vi "timerRunNew.vi"() -> ()   [LabVIEW 2012]
uses:
  <vilib>/addons/database/Connection.llb/DB Tools Open Connec (Path).vi
  <vilib>/addons/database/Connection.llb/Conn Execute.vi
  <vilib>/addons/database/Recordset.llb/Rec Fetch Recordset Data (R).vi
  <vilib>/addons/database/Recordset.llb/Rec Destroy - Connection.vi
  <vilib>/addons/database/_DB Variant To Data/Database Variant To Data.xnode
  <vilib>/addons/database/NI_Database_API.lvlib
panel:
  out "error out 4":errorcluster
  out "error out 3":errorcluster
  out "recordset data 3":variant[][](array[variant])
  out "error out 2":errorcluster
  out "recordset data 2":variant[][](array[variant])
  out "error out":errorcluster
  out "recordset data":variant[][](array[variant])
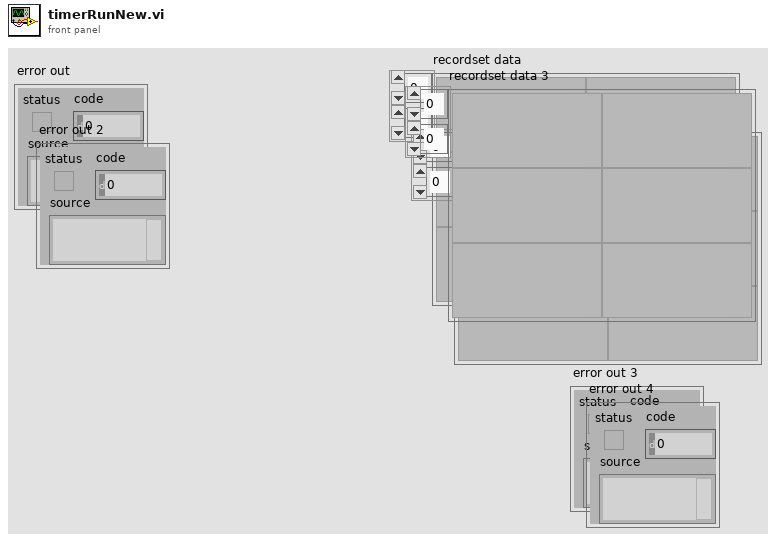
[diagram p1: front panel]
types:
  T1 = typedef "NI_Database_API.lvlib/Conn ObjectReference.ctl" = refnum<k1>
  T2 = typedef "NI_Database_API.lvlib/Rec ObjectReference.ctl" = refnum<k1>
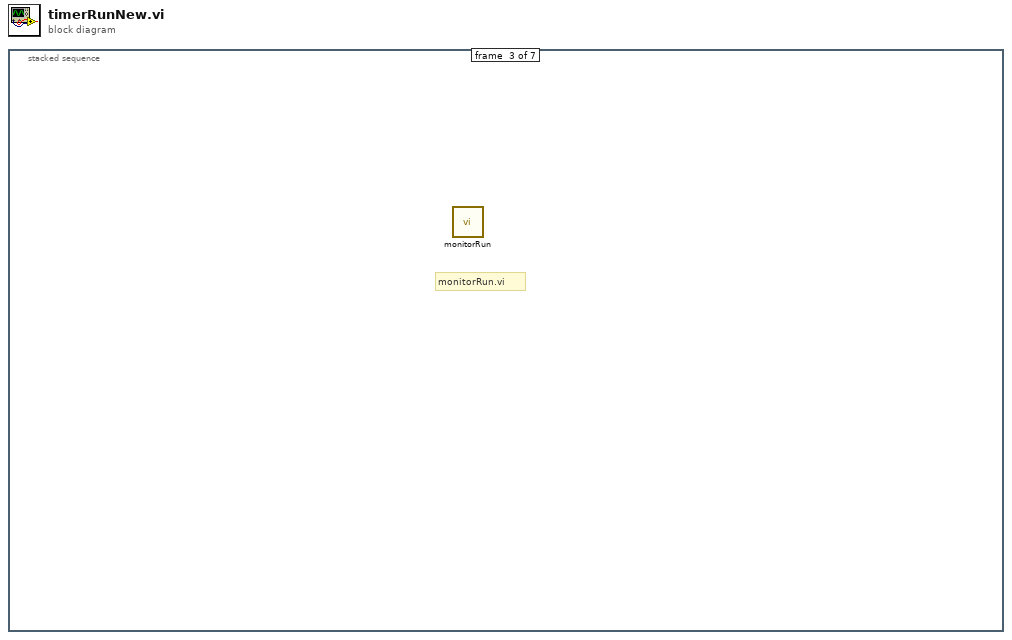
[diagram p0: block diagram]
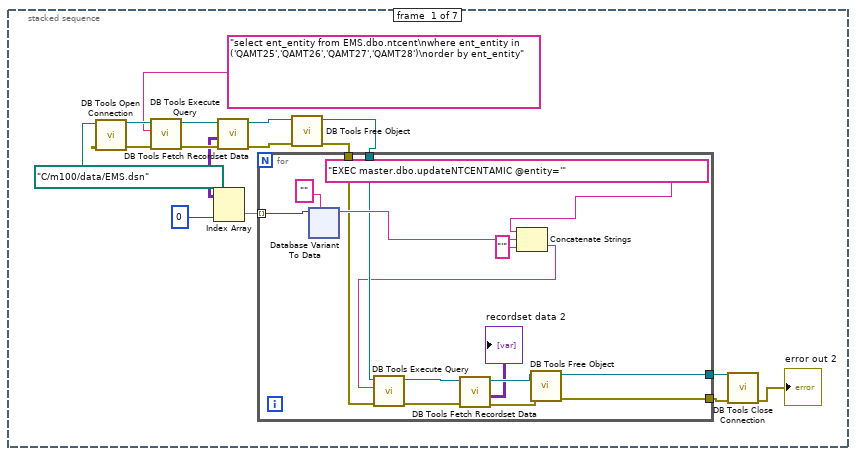
[diagram p2: hidden frame]
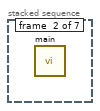
[diagram p3: hidden frame]
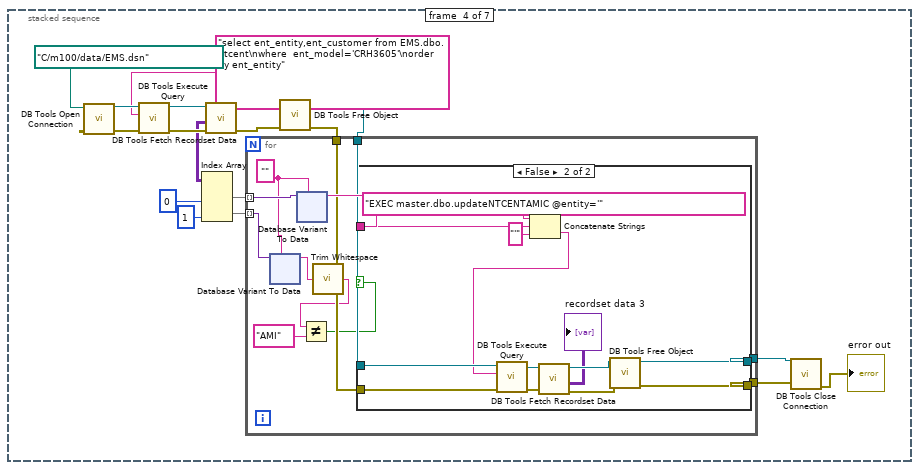
[diagram p4: hidden frame]
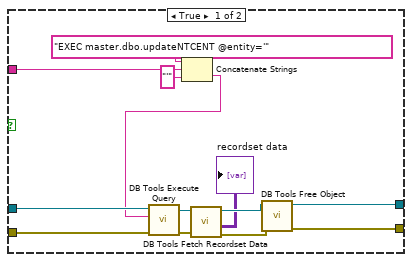
[diagram p5: hidden frame]
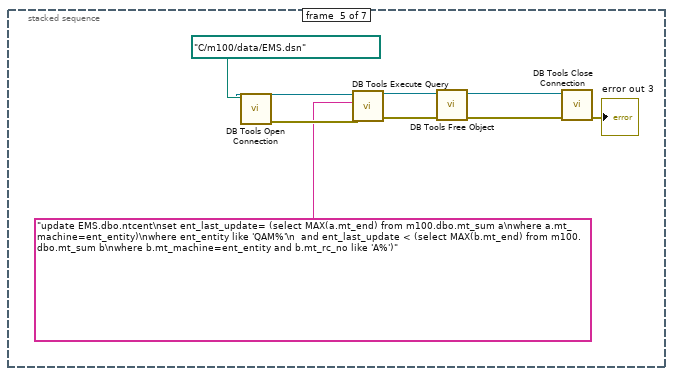
[diagram p6: hidden frame]
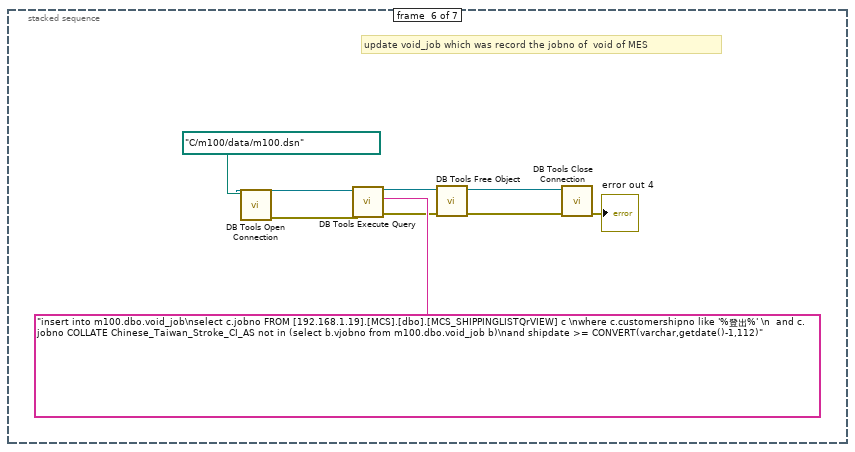
[diagram p7: hidden frame]
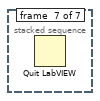
[diagram p8: hidden frame]
diagram:
  n1 = stacked-sequence {
    frame #0 {
      n2 = call-poly <vilib>:"DB Tools Open Connection.vi"("connection information"=path "C:/m100/data/EMS.dsn") -> ("error out"=w1:errorcluster, "connection reference"=w15:T1)  [unwired: 7 in]
      n3 = call-poly <vilib>:"DB Tools Execute Query.vi"("error in (no error)"=w1, "SQL query"="select ent_entity from EMS.dbo.ntcent\nwhere ent_entity in ('QAMT25','QAMT26','QAMT27','QAMT28')\norder by ent_entity", "connection reference"=w15) -> ("error out"=w12:errorcluster, "recordset reference"=w14:T2)  [unwired: 5 in]
      n4 = call-poly <vilib>:"DB Tools Fetch Recordset Data.vi"("error in (no error)"=w12, "recordset reference"=w14) -> ("error out"=w11:errorcluster, "recordset data"=w9:variant[][], "recordset reference out"=w13:T2)  [unwired: 3 in]
      n5 = Index Array(array=w9, index (col)=0 ("disabled index (col)")) -> (element=w7:variant[])  [unwired: 1 in]
      n6 = call-poly <vilib>:"DB Tools Free Object.vi"("error in (no error)"=w11, "recordset reference"=w13) -> ("error out"=w5:errorcluster, "connection reference"=w6:T1)  [unwired: 8 in]
      n7 = for {
        tunnel: w7 -> [w26] mode=indexing
        tunnel: w6 -> [w22]
        tunnel: w5 -> [w21]
        tunnel: [w19] -> w4
        tunnel: [w18] -> w3
        n8 = xnode "Database Variant To Data"("database variant"=w26, "type"="") -> ("data"=w24:string)  [unwired: 1 in, 1 out]
        n9 = Concatenate Strings("EXEC master.dbo.updateNTCENTAMIC @entity='" ("SQL query"), w24, "'" ("string")) -> (w20:string)
        n10 = call-poly <vilib>:"DB Tools Execute Query.vi"("error in (no error)"=w21, "SQL query"=w20, "connection reference"=w22) -> ("error out"=w30:errorcluster, "recordset reference"=w31:T2)  [unwired: 5 in]
        n11 = call-poly <vilib>:"DB Tools Fetch Recordset Data.vi"("error in (no error)"=w30, "recordset reference"=w31) -> ("error out"=w28:errorcluster, "recordset data"=→"recordset data 2":variant[][], "recordset reference out"=w29:T2)  [unwired: 3 in]
        n12 = call-poly <vilib>:"DB Tools Free Object.vi"("error in (no error)"=w28, "recordset reference"=w29) -> ("error out"=w18:errorcluster, "connection reference"=w19:T1)  [unwired: 8 in]
      }
      n13 = call <vilib>:"DB Tools Close Connection.vi"("error in (no error)"=w3, "connection reference"=w4) -> ("error out"=→"error out 2":errorcluster)  [unwired: 5 in]
    }
    frame #1 {
      n14 = call "main.vi"() -> ()  [unwired: 10 in, 1 out]
    }
    frame #2 {
      # "monitorRun.vi"
      n15 = call "monitorRun.vi"() -> ()  [unwired: 12 in]
    }
    frame #3 {
      n16 = call-poly <vilib>:"DB Tools Open Connection.vi"("connection information"=path "C:/m100/data/EMS.dsn") -> ("error out"=w66:errorcluster, "connection reference"=w80:T1)  [unwired: 7 in]
      n17 = call-poly <vilib>:"DB Tools Execute Query.vi"("error in (no error)"=w66, "SQL query"="select ent_entity,ent_customer from EMS.dbo.ntcent\nwhere  ent_model='CRH3605'\norder by ent_entity", "connection reference"=w80) -> ("error out"=w77:errorcluster, "recordset reference"=w79:T2)  [unwired: 5 in]
      n18 = call-poly <vilib>:"DB Tools Fetch Recordset Data.vi"("error in (no error)"=w77, "recordset reference"=w79) -> ("error out"=w76:errorcluster, "recordset data"=w74:variant[][], "recordset reference out"=w78:T2)  [unwired: 3 in]
      n19 = Index Array(array=w74, index (col) #1=0 ("disabled index (col)"), index (col) #2=1 ("index (col)")) -> (element #1=w72:variant[], element #2=w64:variant[])  [unwired: 2 in]
      n20 = call-poly <vilib>:"DB Tools Free Object.vi"("error in (no error)"=w76, "recordset reference"=w78) -> ("error out"=w70:errorcluster, "connection reference"=w71:T1)  [unwired: 8 in]
      n21 = for {
        tunnel: w72 -> [w93] mode=indexing
        tunnel: w71 -> [w91]
        tunnel: w70 -> [w90]
        tunnel: [w89] -> w69
        tunnel: [w88] -> w68
        tunnel: w64 -> [w86] mode=indexing
        w87 = ""
        n22 = xnode "Database Variant To Data"("database variant"=w86, "type"=w87) -> ("data"=w83:string)  [unwired: 1 in, 1 out]
        n23 = xnode "Database Variant To Data"("database variant"=w93, "type"=w87) -> ("data"=w92:string)  [unwired: 1 in, 1 out]
        n24 = call <vilib>:"Trim Whitespace.vi"("string"=w83) -> ("trimmed string"=w82:string)  [unwired: 1 in]
        n25 = Not Equal?(x=w82, y="AMI") -> (x != y?=w84:bool)
        n26 = case shown="False" w84 {
          tunnel: w92 -> [w132 w145]
          tunnel: w91 -> [w130 w143]
          tunnel: w90 -> [w129 w142]
          tunnel: [w127 w140] -> w89
          tunnel: [w126 w139] -> w88
          frame True {
            n27 = Concatenate Strings("EXEC master.dbo.updateNTCENT @entity='" ("SQL query"), w132, "'" ("string")) -> (w128:string)
            n28 = call-poly <vilib>:"DB Tools Execute Query.vi"("error in (no error)"=w129, "SQL query"=w128, "connection reference"=w130) -> ("error out"=w137:errorcluster, "recordset reference"=w138:T2)  [unwired: 5 in]
            n29 = call-poly <vilib>:"DB Tools Fetch Recordset Data.vi"("error in (no error)"=w137, "recordset reference"=w138) -> ("error out"=w135:errorcluster, "recordset data"=→"recordset data":variant[][], "recordset reference out"=w136:T2)  [unwired: 3 in]
            n30 = call-poly <vilib>:"DB Tools Free Object.vi"("error in (no error)"=w135, "recordset reference"=w136) -> ("error out"=w126:errorcluster, "connection reference"=w127:T1)  [unwired: 8 in]
          }
          frame False {
            n31 = Concatenate Strings("EXEC master.dbo.updateNTCENTAMIC @entity='" ("SQL query"), w145, "'" ("string")) -> (w141:string)
            n32 = call-poly <vilib>:"DB Tools Execute Query.vi"("error in (no error)"=w142, "SQL query"=w141, "connection reference"=w143) -> ("error out"=w150:errorcluster, "recordset reference"=w151:T2)  [unwired: 5 in]
            n33 = call-poly <vilib>:"DB Tools Fetch Recordset Data.vi"("error in (no error)"=w150, "recordset reference"=w151) -> ("error out"=w148:errorcluster, "recordset data"=→"recordset data 3":variant[][], "recordset reference out"=w149:T2)  [unwired: 3 in]
            n34 = call-poly <vilib>:"DB Tools Free Object.vi"("error in (no error)"=w148, "recordset reference"=w149) -> ("error out"=w139:errorcluster, "connection reference"=w140:T1)  [unwired: 8 in]
          }
        }
      }
      n35 = call <vilib>:"DB Tools Close Connection.vi"("error in (no error)"=w68, "connection reference"=w69) -> ("error out"=→"error out":errorcluster)  [unwired: 5 in]
    }
    frame #4 {
      n36 = call-poly <vilib>:"DB Tools Open Connection.vi"("connection information"=path "C:/m100/data/EMS.dsn") -> ("error out"=w190:errorcluster, "connection reference"=w191:T1)  [unwired: 7 in]
      n37 = call-poly <vilib>:"DB Tools Execute Query.vi"("error in (no error)"=w190, "SQL query"="update EMS.dbo.ntcent\nset ent_last_update= (select MAX(a.mt_end) from m100.dbo.mt_sum a\nwhere a.mt_machine=ent_entity)\nwhere ent_entity like 'QAM%'\n  and ent_last_update < (select MAX(b.mt_end) from m100.dbo.mt_sum b\nwhere b.mt_machine=ent_entity and b.mt_rc_no like 'A%')", "connection reference"=w191) -> ("error out"=w187:errorcluster, "recordset reference"=w188:T2)  [unwired: 5 in]
      n38 = call-poly <vilib>:"DB Tools Free Object.vi"("error in (no error)"=w187, "recordset reference"=w188) -> ("error out"=w185:errorcluster, "connection reference"=w186:T1)  [unwired: 8 in]
      n39 = call <vilib>:"DB Tools Close Connection.vi"("error in (no error)"=w185, "connection reference"=w186) -> ("error out"=→"error out 3":errorcluster)  [unwired: 5 in]
    }
    frame #5 {
      # "update void_job which was record the jobno of  void of MES"
      n40 = call-poly <vilib>:"DB Tools Open Connection.vi"("connection information"=path "C:/m100/data/m100.dsn") -> ("error out"=w199:errorcluster, "connection reference"=w200:T1)  [unwired: 7 in]
      n41 = call-poly <vilib>:"DB Tools Execute Query.vi"("error in (no error)"=w199, "SQL query"="insert into m100.dbo.void_job\nselect c.jobno FROM [192.168.1.19].[MCS].[dbo].[MCS_SHIPPINGLISTQrVIEW] c \nwhere c.customershipno like '%登出%' \n  and c.jobno COLLATE Chinese_Taiwan_Stroke_CI_AS not in (select b.vjobno from m100.dbo.void_job b)\nand shipdate >= CONVERT(varchar,getdate()-1,112)", "connection reference"=w200) -> ("error out"=w196:errorcluster, "recordset reference"=w197:T2)  [unwired: 5 in]
      n42 = call-poly <vilib>:"DB Tools Free Object.vi"("error in (no error)"=w196, "recordset reference"=w197) -> ("error out"=w194:errorcluster, "connection reference"=w195:T1)  [unwired: 8 in]
      n43 = call <vilib>:"DB Tools Close Connection.vi"("error in (no error)"=w194, "connection reference"=w195) -> ("error out"=→"error out 4":errorcluster)  [unwired: 5 in]
    }
    frame #6 {
      n44 = Quit LabVIEW() -> ()  [unwired: 1 in]
    }
  }
